vi "Fetch Waveforms.vi"(8 "error in":errorcluster, 11 "Rigol DS1054 in":refnum<class "Rigol DS1054.lvclass">) -> (0 "error out":errorcluster, 3 "Rigol DS1054 out":refnum<class "Rigol DS1054.lvclass">)   [LabVIEW 2023, in "RIGOL DS1054.lvlib" / "Rigol DS1054.lvclass"]
uses:
  Rigol DS1054.lvclass
  Scope Base/Scope Base.lvclass/Scope Base.ctl
  Interfaces/IConfigure Scope/IConfigure Scope.lvclass
  Rigol DS1054.lvclass/Rigol DS1054.ctl
  Scope Base/Scope Base.lvclass
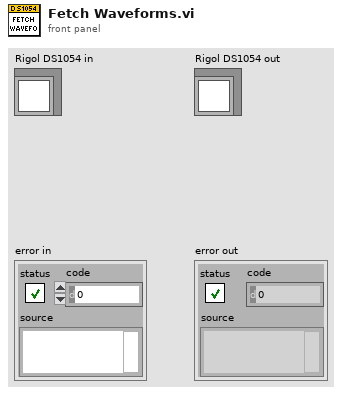
[diagram p1: front panel]
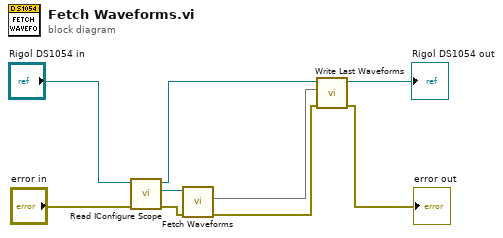
[diagram p0: block diagram]
diagram:
  n1 = call "Read IConfigure Scope.vi"("error in (no error)"="error in", "Scope Base in"="Rigol DS1054 in") -> ("error out"=w4:errorcluster, "IConfigureScope"=w5:refnum<class "IConfigure Scope.lvclass">, "Scope Base out"=w1:refnum<class "Rigol DS1054.lvclass">)  [unwired: 7 in]
  n2 = call-dynamic "Fetch Waveforms.vi"("error in (no error)"=w4, "IConfigure Scope in"=w5) -> ("error out"=w3:errorcluster, "Last Waveforms"=w2:map{u8, waveform(dbl)})  [unwired: 7 in, 1 out]
  n3 = call "Write Last Waveforms.vi"("error in (no error)"=w3, "Last Waveforms"=w2, "Scope Base in"=w1) -> ("error out"=→"error out":errorcluster, "Scope Base out"=→"Rigol DS1054 out":refnum<class "Rigol DS1054.lvclass">)  [unwired: 7 in]
